vi "GetSubarrayFromBufferPOLYMORPHIC.vi"   [LabVIEW 2016]
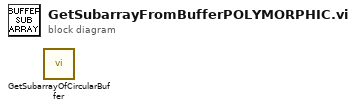
[diagram p0: block diagram]
diagram:
  n1 = call "GetSubarrayOfCircularBuffer.vi"() -> ()  [unwired: 11 in, 1 out]
